vi "Write Context.vi"(8 "error in (no error)":errorcluster, 10 "Context":variant, 11 "HamburgerMenu in":refnum<class "HamburgerMenu.lvclass">) -> (0 "error out":errorcluster, 3 "HamburgerMenu out":refnum<class "HamburgerMenu.lvclass">)   [LabVIEW 2017, in "Hamburger Menu Library.lvlib" / "HamburgerMenu.lvclass"]
uses:
  HamburgerMenu.lvclass
  HamburgerMenu.lvclass/HamburgerMenu.ctl
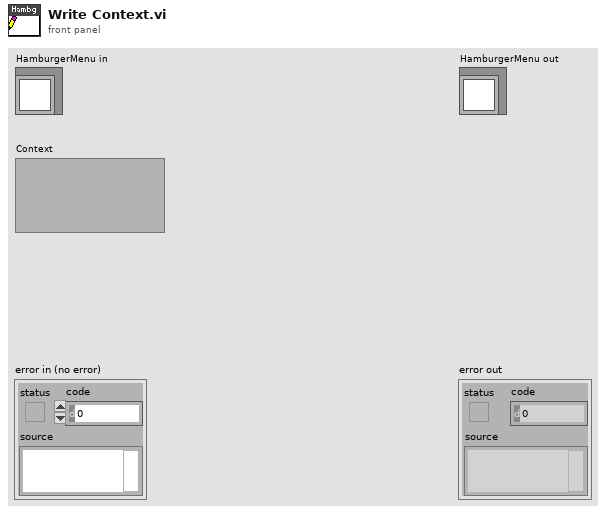
[diagram p1: front panel]
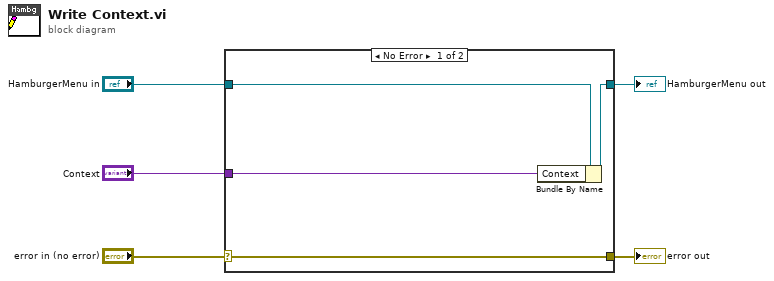
[diagram p0: block diagram]
diagram:
  n1 = case shown="No Error" "error in (no error)" {
    selector: "error in (no error)" -> [w9 w10]
    tunnel: [w9 w10] -> w4
    tunnel: [w7 w11] -> w2
    tunnel: "HamburgerMenu in" -> [w8 w11]
    tunnel: "Context" -> [w6 _]
    frame No Error {
      n2 = Bundle By Name(cluster=w8, "Context"=w6) -> (w7:refnum<class "HamburgerMenu.lvclass">)
    }
    frame Error {
    }
  }
  "error out" <- w4
  "HamburgerMenu out" <- w2
